vi "OTP - Generate Key.vi"(11 "Length":i32) -> (3 "key (Private)":string)   [LabVIEW 2013]
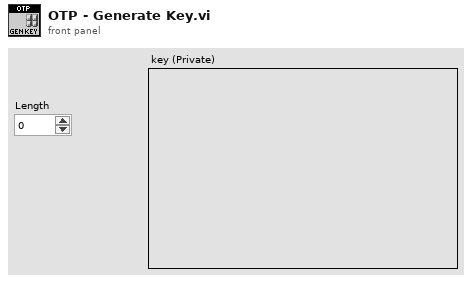
[diagram p1: front panel]
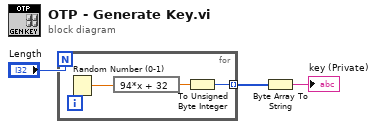
[diagram p0: block diagram]
diagram:
  n1 = for {
    N: "Length" -> [_]
    tunnel: [w4] -> w1 mode=indexing
    n2 = Random Number (0-1)() -> (number: 0 to 1=w6:dbl)
    n3 = expression code="94*x + 32"(w6) -> (w5:dbl)
    n4 = To Unsigned Byte Integer(number=w5) -> (unsigned 8bit integer=w4:u8)
  }
  n5 = Byte Array To String(unsigned byte array=w1) -> (string=→"key (Private)":string)
